vi "Get SLSC Switch Switches JSON.vi"(8 "error in":errorcluster, 11 "slsc switch custom device in":T1 format="%.0x") -> (0 "error out":errorcluster, 2 "switches json":string, 3 "slsc switch custom device out":T1 format="%.0x")   [LabVIEW 2017, in "SLSC Switch Scripting.lvlib"]
doc: "Returns the JSON string set by using <b>Load SLSC Switch Module Configuration.vi</b> or <b>Autodetect SLSC Switch Module Configuration.vi</b>."
uses:
  SLSC Switch Scripting.lvlib
  <vilib>/NI Veristand/Custom Device API/Custom Device Item Ref.ctl
  SLSC Scripting Constants.vi
  <vilib>/NI Veristand/Custom Device API/Get Item Property (String).vi
  <vilib>/NI Veristand/Custom Device API/Custom Device API.lvlib
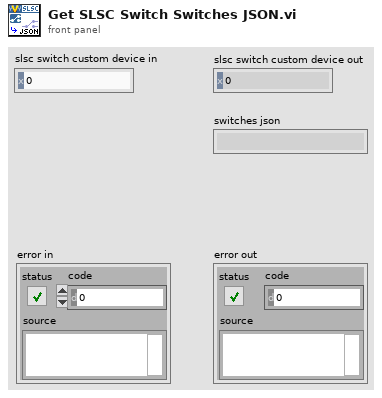
[diagram p1: front panel]
types:
  T1 = typedef "Custom Device API.lvlib/Custom Device Item Ref.ctl" = u64
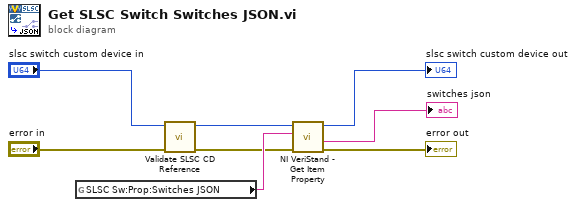
[diagram p0: block diagram]
diagram:
  n1 = global read "SLSC Scripting Constants.vi" "SLSC Sw:Prop:Switches JSON"() -> (w6:string)
  n2 = call "Validate SLSC CD Reference.vi"("error in"="error in", "slsc switch custom device in"="slsc switch custom device in") -> ("error out"=w3:errorcluster, "slsc switch custom device out"=w2:T1)  [unwired: 8 in]
  n3 = call-poly <vilib>:"NI VeriStand - Get Item Property.vi"("error in (no error)"=w3, "Property Name"=w6, "Item Ref in"=w2) -> ("error out"=→"error out":errorcluster, "Value"=→"switches json":string, "Item Ref out"=→"slsc switch custom device out":T1)  [unwired: 5 in, 1 out]
